vi "getPressure.vi"(6 "Channel":i32, 8 "error in (no error)":errorcluster, 11 "Instrument.Cryostat in":refnum<class "Instrument.Cryostat.lvclass">) -> (0 "error out":errorcluster, 1 "Status":string, 2 "Pressure (mbar)":dbl, 3 "Instrument.Cryostat out":refnum<class "Instrument.Cryostat.lvclass">)   [LabVIEW 2019, in "Instrument.Cryostat.lvclass"]
uses:
  Instrument.Cryostat.lvclass
  Instrument/Instrument.lvclass
  8735d4ed-0b7a-46cb-9742-e560619e7b60.vi
  Typedefs/getPressure--cluster.ctl
  C:/Users/patrick/Documents/GitHub/Instrument-Framework/lvsrc/Instrument/Instrument.lvclass
  C:/Program Files (x86)/National Instruments/LabVIEW 2019/vi.lib/JKI/JKI SMO/SMO/SMO.lvclass
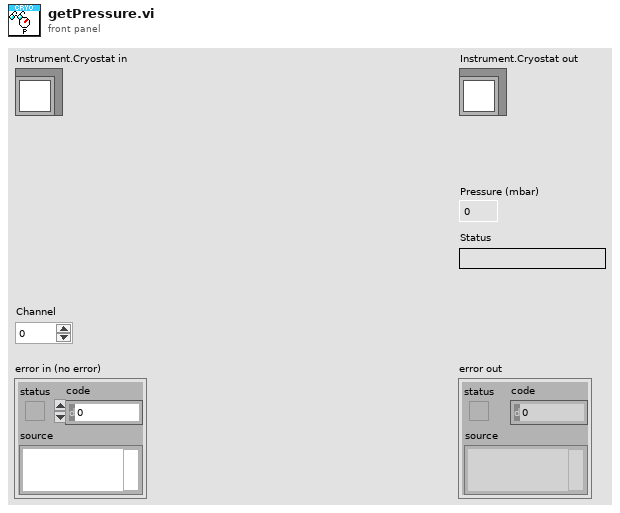
[diagram p1: front panel]
types:
  T1 = typedef "Instrument.Cryostat.lvclass/getPressure--cluster.ctl" = cluster{"Pressure":dbl, "Status":string}
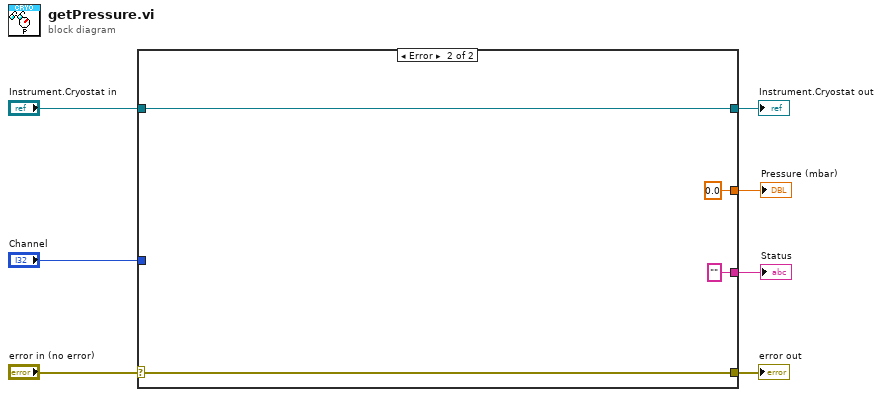
[diagram p0: block diagram]
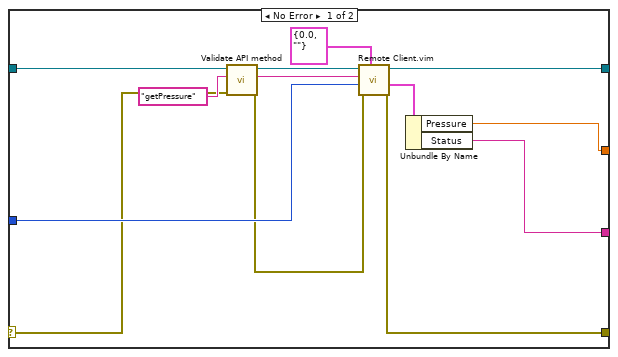
[diagram p2: hidden frame]
diagram:
  n1 = case shown="Error" "error in (no error)" {
    selector: "error in (no error)" -> [w14 w24]
    tunnel: [w12 w24] -> w6
    tunnel: [w16 w23] -> w4
    tunnel: "Instrument.Cryostat in" -> [w17 w23]
    tunnel: "Channel" -> [w15 _]
    tunnel: [w9 0.0 ("Pressure")] -> w2
    tunnel: [w8 "" ("Status")] -> w1
    frame No Error {
      n2 = call "Validate API method.vi"("error in (no error)"=w14, "command in"="getPressure" ("error message (\"\")"), "Instrument in"=w17) -> ("error out"=w13:errorcluster, "command out"=w19:string, "Instrument out"=w18:refnum<class "Instrument.Cryostat.lvclass">)  [unwired: 6 in]
      n3 = call "Remote Client.vim"("Data Out type"=T1 {"Pressure"=0.0, "Status"=""} ("getPressure"), "error in (no error)"=w13, "params"=w15, "method"=w19, "Instrument in"=w18) -> ("error out"=w12:errorcluster, "Data out"=w10:T1, "Instrument out"=w16:refnum<class "Instrument.Cryostat.lvclass">)  [unwired: 3 in, 1 out]
      n4 = Unbundle By Name(w10) -> ("Pressure"=w9:dbl, "Status"=w8:string)
    }
    frame Error {
    }
  }
  "error out" <- w6
  "Instrument.Cryostat out" <- w4
  "Pressure (mbar)" <- w2
  "Status" <- w1
